vi "SetButtonDefinitionFile.vi"(8 "Error In":errorcluster, 10 "ButtonDefinitionFile":string, 11 "reference in":refnum<class "VerticalButtonBar.lvclass">) -> (0 "Error Out":errorcluster, 3 "reference in":refnum<class "VerticalButtonBar.lvclass">)   [LabVIEW 2021, in "VerticalButtonBar.lvclass"]
uses:
  VerticalButtonBar.lvclass
  ButtonCollection/ButtonCollection.lvclass
  .Externals/Library_TAF_ApplicationFramework/Application/Application.lvclass
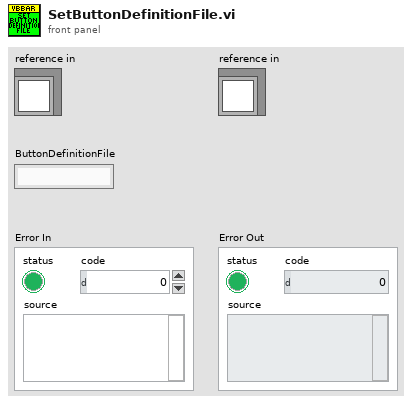
[diagram p1: front panel]
types:
  T1 = typedef "VerticalButtonBar.lvclass/ObjectAttributes.ctl" = cluster{"Interfaces":cluster{"IDockGUI":refnum<class "IDockGUI.lvclass">, "Authorizer":refnum<class "IAuthorization.lvclass">}, "Locals":cluster{"ButtonBar":refnum<class "ButtonCollection.lvclass">, "BaseConfigurationPath":path, "Labels":cluster{"Label":string, "Value":string}[]}, "Persistent":cluster{"ButtonDefinitionFile":string}}
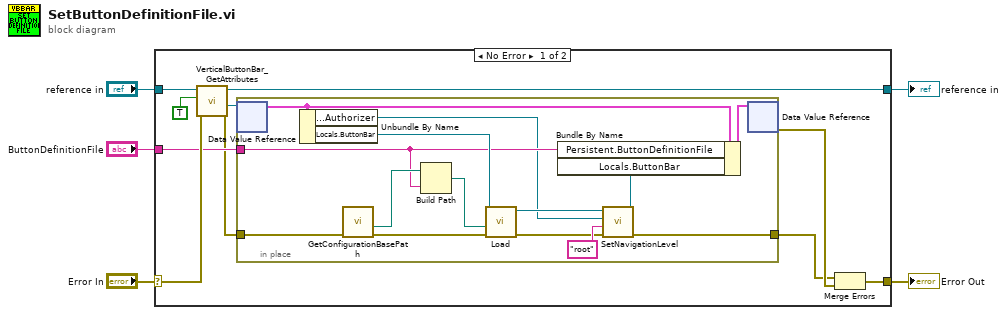
[diagram p0: block diagram]
diagram:
  n1 = case shown="No Error" "Error In" {
    selector: "Error In" -> [w15 w31]
    tunnel: [w13 w31] -> w4
    tunnel: [w11 w30] -> w2
    tunnel: "reference in" -> [w12 w30]
    tunnel: "ButtonDefinitionFile" -> [w8 _]
    frame No Error {
      n2 = call "VerticalButtonBar_GetAttributes.vi"("error in (no error)"=w15, "OnlyGetDvrReference(False)"=TRUE, "reference in"=w12) -> ("error out"=w7:errorcluster, "DataRef"=w9:refnum<data-value>, "reference out"=w11:refnum<class "VerticalButtonBar.lvclass">)  [unwired: 5 in, 1 out]
      n3 = in-place {
        in-place-border: w8 -> [w20]
        in-place-border: w7 -> [w23]
        in-place-border: [w26] -> w6
        n4 = in-place-dvr #1(w9) -> (w28:T1)  [unwired: 1 out]
        n5 = Unbundle By Name(w28) -> ("Interfaces.Authorizer"=w16:refnum<class "IAuthorization.lvclass">, "Locals.ButtonBar"=w27:refnum<class "ButtonCollection.lvclass">)
        n6 = call "GetConfigurationBasePath.vi"("Error In"=w23) -> ("Error Out"=w22:errorcluster, "BasePath"=w21:path)  [unwired: 9 in]
        n7 = Build Path(base path=w21, name or relative path=w20) -> (appended path=w19:path)
        n8 = call "Load.vi"("ErrorIn"=w22, "Path"=w19, "ObjectIn"=w27) -> ("ErrorOut"=w18:errorcluster, "ObjectOut"=w17:refnum<class "ButtonCollection.lvclass">)  [unwired: 7 in]
        n9 = call-dynamic "SetNavigationLevel.vi"("ErrorIn"=w18, "NavigationName"="root", "Authorization"=w16, "ObjectIn"=w17) -> ("ErrorOut"=w26:errorcluster, "ObjectOut"=w24:refnum<class "ButtonCollection.lvclass">)  [unwired: 6 in]
        n10 = Bundle By Name(cluster=w28, "Persistent.ButtonDefinitionFile"=w20, "Locals.ButtonBar"=w24) -> (w29:T1)
        n11 = in-place-dvr #1(w29) -> (w14:errorcluster)  [unwired: 1 out]
      }
      n12 = Merge Errors(w6, w14) -> (w13:errorcluster)
    }
    frame Error {
    }
  }
  "Error Out" <- w4
  "reference in" <- w2
